vi "Test_PowerRequest.vi"(8 "error in (no error)":errorcluster) -> (0 "error out":errorcluster)   [LabVIEW 2020]
doc: "Windows service power request to prevent the computer to go into hybernate if data is logged for a long time."
uses:
  Power Availabilty Requests/Type Defs/Power Request Type.ctl
  Power Availabilty Requests/Type Defs/Test_PR_typedef.ctl
  Power Requests.lvlib
  Builds/Sgraph_lib_V1.lvlib
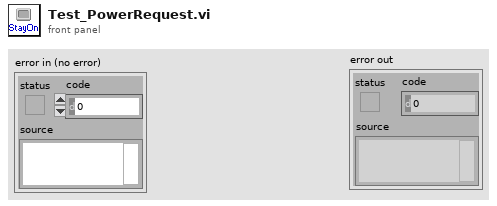
[diagram p1: front panel]
types:
  T1 = typedef "Sgraph_lib_V1.lvlib/Test_PR_typedef.ctl" = enum16{"Start-Allways-ON", "Read-handle"}
  T2 = typedef "Power Requests.lvlib/Power Request Type.ctl" = enum32{"Power Request Display Required", "Power Request System Required", "Power Request Away Mode Required", "Power Request Execution Required"}
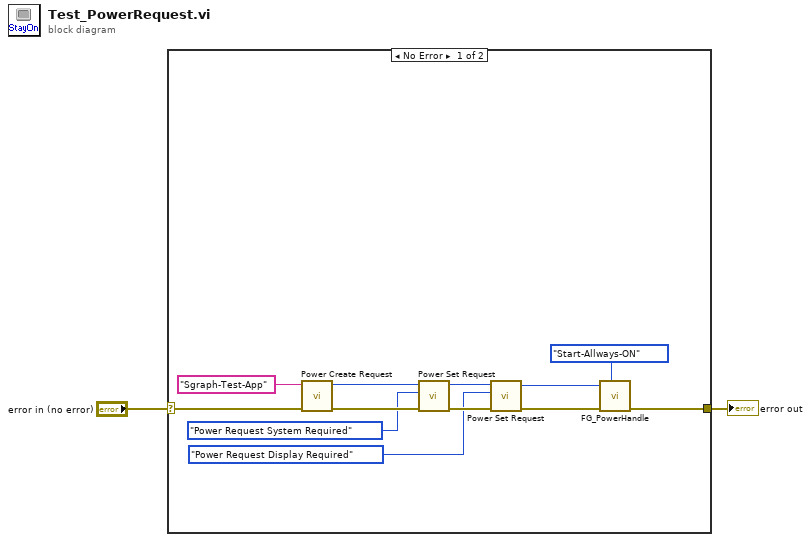
[diagram p0: block diagram]
diagram:
  n1 = case shown="No Error" "error in (no error)" {
    selector: "error in (no error)" -> [w11 w15]
    tunnel: [w3 w15] -> w1
    frame No Error {
      n2 = call "Power Create Request.vi"("error in (no error)"=w11, "Simple Reason String"="Sgraph-Test-App") -> ("error out"=w14:errorcluster, "Handle"=w13:i64)  [unwired: 8 in]
      n3 = call "Power Set Request.vi"("error in (no error)"=w14, "Power Request Type"=Power_Request_Type."Power Request System Required", "Handle in"=w13) -> ("error out"=w9:errorcluster, "Handle out"=w5:u32)  [unwired: 6 in, 1 out]
      n4 = call "Power Set Request.vi"("error in (no error)"=w9, "Power Request Type"=Power_Request_Type."Power Request Display Required", "Handle in"=w5) -> ("error out"=w4:errorcluster, "Handle out"=w6:u32)  [unwired: 6 in, 1 out]
      n5 = call "FG_PowerHandle.vi"("Enum"=Test_PR_typedef."Start-Allways-ON", "error in (no error)"=w4, "Handle in"=w6) -> ("error out"=w3:errorcluster)  [unwired: 7 in, 1 out]
    }
    frame Error {
    }
  }
  "error out" <- w1
